vi "week06_Ex01.vi"() -> ()   [LabVIEW 2017]
panel:
  out "All RND Num":u8[](array[numeric])
  out "Max Value":u8
  out "Max Num":dbl
  out "RND Number":u8
  out "Xi":i32
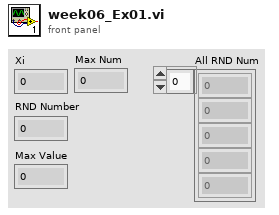
[diagram p1: front panel]
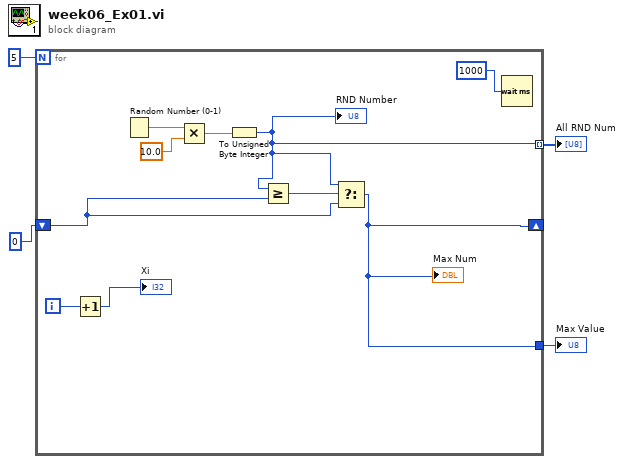
[diagram p0: block diagram]
diagram:
  n1 = for {
    N: 5 -> [_]
    shift-right: [w6] -> _
    shift-left: 0 -> [w8]
    tunnel: [w6] -> w2
    tunnel: [w5] -> w1 mode=indexing
    i -> [w14]
    n2 = Increment(x=w14) -> (x+1=→"Xi":i32)
    n3 = Random Number (0-1)() -> (number: 0 to 1=w11:dbl)
    n4 = Multiply(x=w11, y=10.0) -> (x*y=w9:dbl)
    n5 = To Unsigned Byte Integer(number=w9) -> (unsigned 8bit integer=w5:u8)
    "RND Number" <- w5
    n6 = Greater Or Equal?(x=w5, y=w8) -> (x >= y?=w7:bool)
    n7 = Select(t=w5, s=w7, f=w8) -> (s? t:f=w6:i32)
    "Max Num" <- w6
    n8 = Wait (ms)(milliseconds to wait=u32 1000) -> ()  [unwired: 1 out]
  }
  "Max Value" <- w2
  "All RND Num" <- w1
